vi "biassubsequence1.vi"(0 "diag(J'J)":T1, 1 "frequency":dbl=100.0, 5 "J'J":T1, 7 "delta":dbl=1.0, 9 "J'(y-f(t))":dbl[](array[numeric]) format="%.2f", 11 "y":dbl[](array[numeric]) format="%.2f", 12 "B old":dbl[](array[numeric])) -> (6 "error":dbl, 10 "B new":dbl[](array[numeric]))   [LabVIEW 2021]
uses:
  <vilib>/Analysis/Matrix/Datatypes/RealMatrix.ctl
  <vilib>/Analysis/7linalg.llb/Solve Linear Equations (single right hand).vi
  <vilib>/Analysis/baseanly.llb/Solve Linear Equations By Cholesky.vi
  <vilib>/Analysis/baseanly.llb/Real Matrix to Compact Array.vi
  <vilib>/Analysis/baseanly.llb/Real Compact Tri-Matrix Linear Eqs.vi
  <vilib>/Analysis/Matrix/Numeric/Multiply/Multiply - RM,R.vi
  <vilib>/Analysis/Matrix/Numeric/Add/Add - RM,RM.vi
  <vilib>/Analysis/7linalg.llb/Solve Linear Eqs (General).vi
  <vilib>/Analysis/7linalg.llb/Solve Linear Eqs (Gen, single right hand).vi
  <vilib>/Analysis/NI_AALPro.lvlib
  <vilib>/Analysis/Matrix/NI_Matrix.lvlib
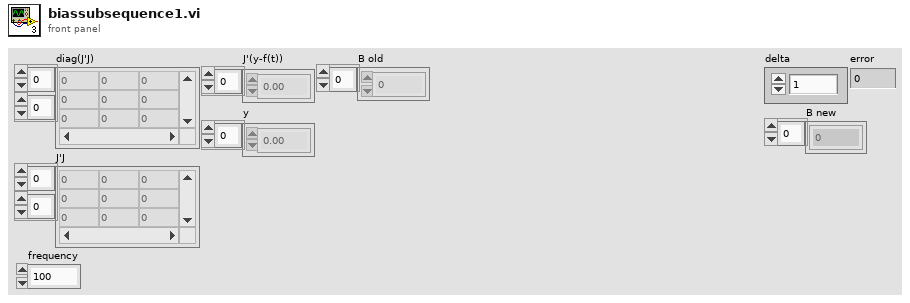
[diagram p1: front panel]
types:
  T1 = typedef "NI_Matrix.lvlib/RealMatrix.ctl" = dbl[][]
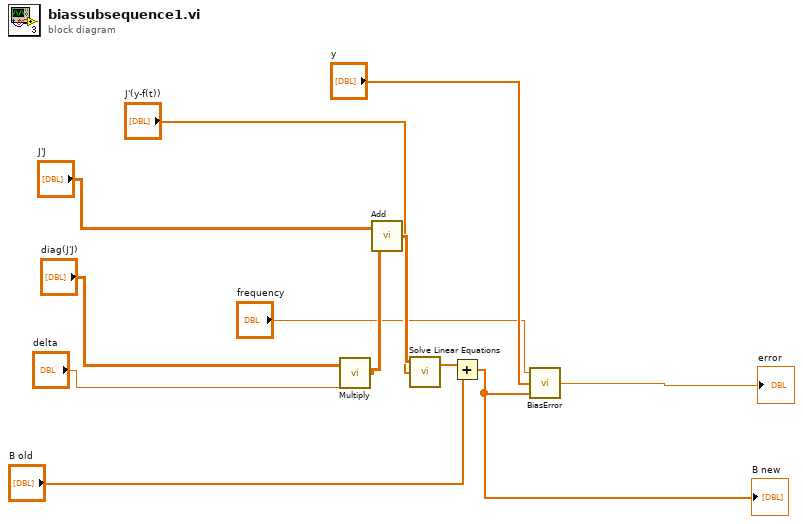
[diagram p0: block diagram]
diagram:
  n1 = call-poly <vilib>:"Multiply.vi"("Real Scalar c"="delta", "Real Matrix A"="diag(J'J)") -> ("A * c"=w12:T1)
  n2 = call-poly <vilib>:"Add.vi"("Real Matrix B"=w12, "Real Matrix A"="J'J") -> ("A + B"=w11:T1)
  n3 = call-poly <vilib>:"Solve Linear Equations.vi"("Known Vector"="J'(y-f(t))", "Input Matrix"=w11) -> ("Solution Vector"=w9:dbl[])  [unwired: 1 in, 1 out]
  n4 = Add(x=w9, y="B old") -> (x+y=w10:dbl[])
  "B new" <- w10
  n5 = call "BiasError.vi"("B"=w10, "y"="y", "frequency"="frequency") -> ("error"=→"error":dbl)
